vi "KE622x -- Get Op Event Reg State.vi"(0 "VISA Resource In":refnum<visa-resource-name>, 1 "Error Query (T)?":bool=TRUE, 11 "error in (no error)":errorcluster) -> (4 "VISA Resource Out (dupl)":refnum<visa-resource-name>, 8 "KE622x Op Event Reg":T1, 15 "error out":errorcluster)   [LabVIEW 2019, in "Keithley 622x.lvlib"]
doc: "Returns the bits in the 'Operation Event' register of the Status Model. Note that only the used (named) bits are returned."
uses:
  Keithley 622x.lvlib
  Typedefs/KE622x -- Op Event Reg State.ctl
panel:
  out "Reg Num (dec)":u16 format="%0d"
  out "Reg Num (binary)":u16 format="%016b"
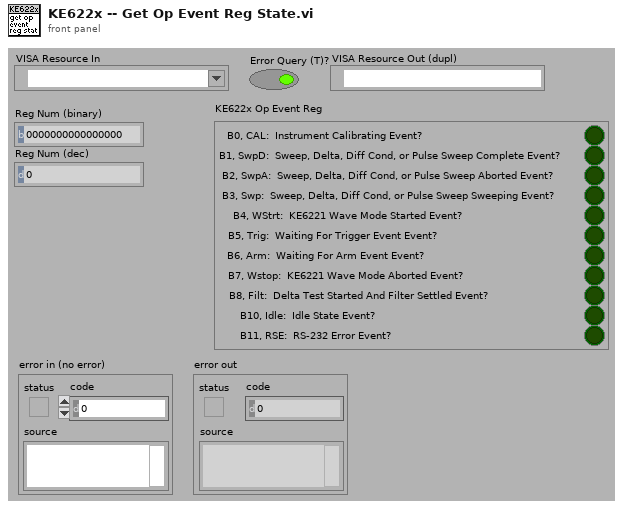
[diagram p1: front panel]
types:
  T1 = typedef "Keithley 622x.lvlib/KE622x -- Op Event Reg State.ctl" = cluster{"B0, CAL:  Instrument Calibrating Event?":bool, "B1, SwpD:  Sweep, Delta, Diff Cond, or Pulse Sweep Complete Event?":bool, "B2, SwpA:  Sweep, Delta, Diff Cond, or Pulse Sweep Aborted Event?":bool, "B3, Swp:  Sweep, Delta, Diff Cond, or Pulse Sweep Sweeping Event?":bool, "B4, WStrt:  KE6221 Wave Mode Started Event?":bool, "B5, Trig:  Waiting For Trigger Event Event?":bool, "B6, Arm:  Waiting For Arm Event Event?":bool, "B7, Wstop:  KE6221 Wave Mode Aborted Event?":bool, "B8, Filt:  Delta Test Started And Filter Settled Event?":bool, "B10, Idle:  Idle State Event?":bool, "B11, RSE:  RS-232 Error Event?":bool}
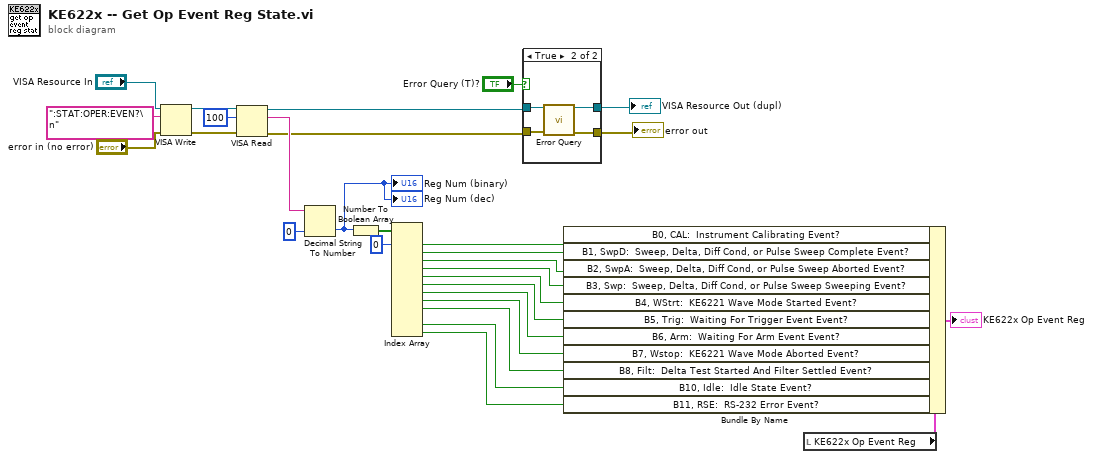
[diagram p0: block diagram]
diagram:
  n1 = VISA Write(VISA resource name="VISA Resource In", write buffer=":STAT:OPER:EVEN?\n", error in (no error)="error in (no error)") -> (VISA resource name out=w26:refnum<visa-resource-name>, error out=w25:errorcluster)  [unwired: 1 out]
  n2 = VISA Read(VISA resource name=w26, byte count=u32 100, error in (no error)=w25) -> (VISA resource name out=w16:refnum<visa-resource-name>, read buffer=w23:string, error out=w17:errorcluster)  [unwired: 1 out]
  n3 = Decimal String To Number(string=w23, default (0L)=u16 0 ("default (0 I32)")) -> (number=w18:u16)  [unwired: 2 out]
  "Reg Num (binary)" <- w18
  "Reg Num (dec)" <- w18
  n4 = Number To Boolean Array(number=w18) -> (Boolean array=w21:bool[])
  n5 = Index Array(array=w21, index #1=0 ("index")) -> (element #1=w12:bool, element #2=w11:bool, element #3=w10:bool, element #4=w9:bool, element #5=w8:bool, element #6=w7:bool, element #7=w6:bool, element #8=w5:bool, element #9=w4:bool, element #11=w3:bool, element #12=w2:bool)  [unwired: 11 in, 1 out]
  n6 = case shown="True" "Error Query (T)?" {
    tunnel: w17 -> [w30 w35]
    tunnel: w16 -> [w31 w34]
    tunnel: [w30 w33] -> w14
    tunnel: [w31 w32] -> w15
    frame False {
    }
    frame True {
      n7 = call "Error Query.vi"("VISA Resource In"=w34, "error in (no error)"=w35) -> ("VISA Resource Out (dupl)"=w32:refnum<visa-resource-name>, "error out"=w33:errorcluster)  [unwired: 10 in, 2 out]
    }
  }
  "VISA Resource Out (dupl)" <- w15
  "error out" <- w14
  n8 = local read "KE622x Op Event Reg"() -> (w19:T1)
  n9 = Bundle By Name(cluster=w19, "B0, CAL:  Instrument Calibrating Event?"=w12, "B1, SwpD:  Sweep, Delta, Diff Cond, or Pulse Sweep Complete Event?"=w11, "B2, SwpA:  Sweep, Delta, Diff Cond, or Pulse Sweep Aborted Event?"=w10, "B3, Swp:  Sweep, Delta, Diff Cond, or Pulse Sweep Sweeping Event?"=w9, "B4, WStrt:  KE6221 Wave Mode Started Event?"=w8, "B5, Trig:  Waiting For Trigger Event Event?"=w7, "B6, Arm:  Waiting For Arm Event Event?"=w6, "B7, Wstop:  KE6221 Wave Mode Aborted Event?"=w5, "B8, Filt:  Delta Test Started And Filter Settled Event?"=w4, "B10, Idle:  Idle State Event?"=w3, "B11, RSE:  RS-232 Error Event?"=w2) -> (→"KE622x Op Event Reg":T1)
